vi "RTM SLSC DisableEnable.vi"(8 "error in (no error)":errorcluster, 11 "Node Ptr":T1=18446744073709551615 format="%.0x") -> (0 "error out":errorcluster)   [LabVIEW 2019, in "SLSC EDS System Explorer.lvlib"]
uses:
  SLSC EDS System Explorer.lvlib
  <vilib>/NI VeriStand/Custom Device API/Custom Device Item Ref.ctl
  Shared/Constants.vi
  <vilib>/NI VeriStand/Custom Device API/Custom Device API.lvlib
  Shared/SLSC EDS Shared.lvlib
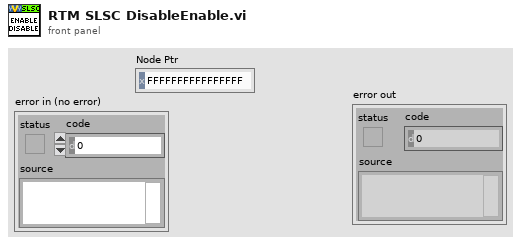
[diagram p1: front panel]
types:
  T1 = typedef "Custom Device API.lvlib/Custom Device Item Ref.ctl" = u64
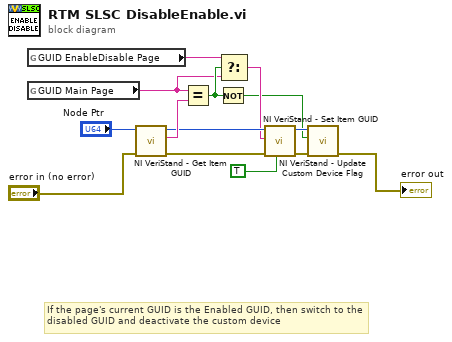
[diagram p0: block diagram]
diagram:
  # "If the page's current GUID is the Enabled GUID, then switch to the disabled GUID and deactivate the custom device"
  n1 = global read "Constants.vi" "GUID EnableDisable Page"() -> (w3:string)
  n2 = global read "Constants.vi" "GUID Main Page"() -> (w4:string)
  n3 = call <vilib>:"NI VeriStand - Get Item GUID.vi"("error in (no error)"="error in (no error)", "Item Ref in"="Node Ptr") -> ("error out"=w11:errorcluster, "GUID"=w13:string, "Item Ref out"=w8:T1)  [unwired: 7 in]
  n4 = Equal?(x=w4, y=w13) -> (x = y?=w5:bool)
  n5 = Not(x=w5) -> (.not. x?=w6:bool)
  n6 = Select(t=w3, s=w5, f=w4) -> (s? t:f=w7:string)
  n7 = call <vilib>:"NI VeriStand - Set Item GUID.vi"("Refresh System Explorer Tree? (F)"=TRUE, "error in (no error)"=w11, "GUID"=w7, "Item Ref in"=w8) -> ("error out"=w10:errorcluster, "Item Ref out"=w9:T1)  [unwired: 6 in]
  n8 = call <vilib>:"NI VeriStand - Update Custom Device Flag.vi"("error in (no error)"=w10, "Is Custom Device Active?"=w6, "Device Ref in"=w9) -> ("error out"=→"error out":errorcluster)  [unwired: 7 in, 1 out]
